vi "VI Tree.vi"   [LabVIEW 2017, in "Agilent E4980.lvlib"]
doc: "This is the instrument driver for the Agilent E4980. The VI Tree displays all the user-callable VIs of the instrument driver in an organized table."
uses:
  Agilent E4980.lvlib
  Action-Status/Clear Comparator Bin (Limit).vi
  Utility/Configure System (Display).vi
  Data/Low Level/Read Functional Data (AC Monitor).vi
panel:
  # "(c) 2007-2015 National Instruments.  ALL RIGHTS RESERVED."
  # "SEE DIAGRAM\nFOR VI TREE."
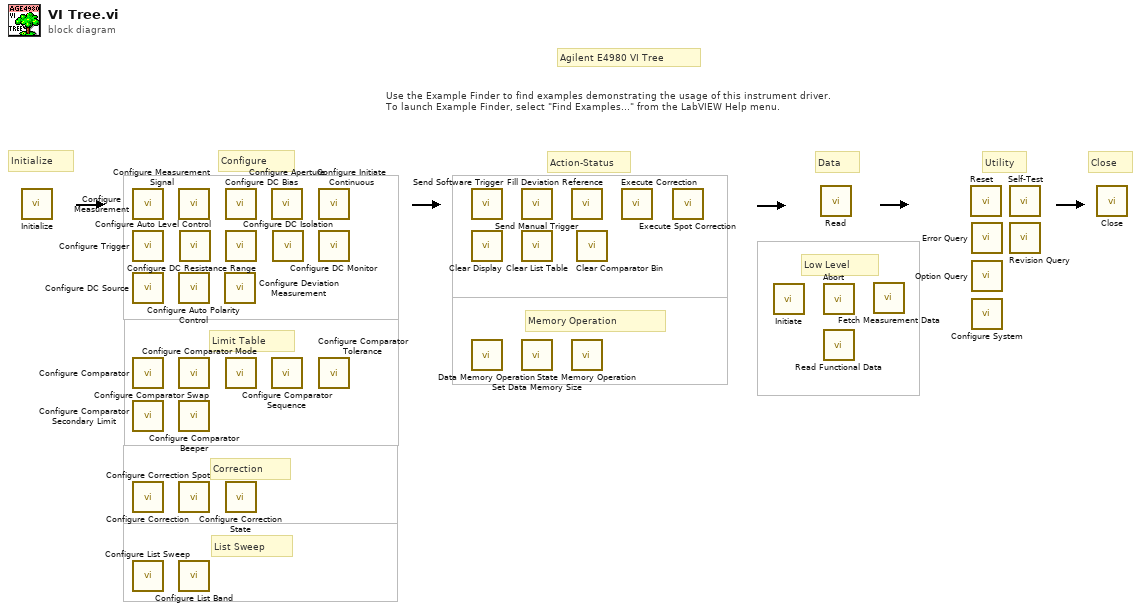
[diagram p0: block diagram]
diagram:
  # "Data"
  # "Low Level"
  # "Memory Operation"
  # "List Sweep"
  # "Correction"
  # "Limit Table"
  # "Close"
  # "Utility"
  # "Action-Status"
  # "Configure"
  # "Initialize"
  # "Agilent E4980 VI Tree"
  # "Use the Example Finder to find examples demonstrating the usage of this instrument driver.\nTo launch Example Finder, select \"Find Examples...\" from the LabVIEW Help menu."
  n1 = call "Initialize.vi"() -> ()  [unwired: 10 in, 2 out]
  n2 = call "Configure Measurement.vi"() -> ()  [unwired: 10 in, 2 out]
  n3 = call "Configure Trigger.vi"() -> ()  [unwired: 10 in, 2 out]
  n4 = call "Configure DC Source.vi"() -> ()  [unwired: 10 in, 2 out]
  n5 = call "Configure Comparator.vi"() -> ()  [unwired: 10 in, 2 out]
  n6 = call "Configure Comparator Secondary Limit.vi"() -> ()  [unwired: 10 in, 2 out]
  n7 = call "Configure Correction.vi"() -> ()  [unwired: 10 in, 2 out]
  n8 = call "Configure List Sweep.vi"() -> ()  [unwired: 10 in, 2 out]
  n9 = call "Configure Measurement Signal.vi"() -> ()  [unwired: 10 in, 2 out]
  n10 = call "Configure Auto Polarity Control.vi"() -> ()  [unwired: 10 in, 2 out]
  n11 = call "Configure Comparator Swap.vi"() -> ()  [unwired: 10 in, 2 out]
  n12 = call "Configure Comparator Beeper.vi"() -> ()  [unwired: 10 in, 2 out]
  n13 = call "Configure Correction Spot.vi"() -> ()  [unwired: 10 in, 2 out]
  n14 = call "Configure List Band.vi"() -> ()  [unwired: 10 in, 2 out]
  n15 = call "Configure Auto Level Control.vi"() -> ()  [unwired: 10 in, 2 out]
  n16 = call "Configure Deviation Measurement.vi"() -> ()  [unwired: 10 in, 2 out]
  n17 = call "Configure DC Bias.vi"() -> ()  [unwired: 10 in, 2 out]
  n18 = call "Configure DC Resistance Range.vi"() -> ()  [unwired: 10 in, 2 out]
  n19 = call "Configure Comparator Mode.vi"() -> ()  [unwired: 10 in, 2 out]
  n20 = call "Configure Correction State.vi"() -> ()  [unwired: 10 in, 2 out]
  n21 = call "Configure Aperture.vi"() -> ()  [unwired: 10 in, 2 out]
  n22 = call "Configure Comparator Sequence.vi"() -> ()  [unwired: 10 in, 2 out]
  n23 = call "Configure DC Isolation.vi"() -> ()  [unwired: 10 in, 2 out]
  n24 = call "Configure Initiate Continuous.vi"() -> ()  [unwired: 10 in, 2 out]
  n25 = call "Configure DC Monitor.vi"() -> ()  [unwired: 10 in, 2 out]
  n26 = call "Configure Comparator Tolerance.vi"() -> ()  [unwired: 10 in, 2 out]
  n27 = call "Send Software Trigger.vi"() -> ()  [unwired: 10 in, 2 out]
  n28 = call "Clear Display.vi"() -> ()  [unwired: 10 in, 2 out]
  n29 = call "Data Memory Operation.vi"() -> ()  [unwired: 10 in, 2 out]
  n30 = call "Send Manual Trigger.vi"() -> ()  [unwired: 10 in, 2 out]
  n31 = call "Clear List Table.vi"() -> ()  [unwired: 10 in, 2 out]
  n32 = call "Set Data Memory Size.vi"() -> ()  [unwired: 10 in, 2 out]
  n33 = call "Fill Deviation Reference.vi"() -> ()  [unwired: 10 in, 2 out]
  n34 = call "State Memory Operation.vi"() -> ()  [unwired: 10 in, 2 out]
  n35 = call-poly "Clear Comparator Bin.vi"() -> ()  [unwired: 10 in, 2 out]
  n36 = call "Execute Correction.vi"() -> ()  [unwired: 10 in, 2 out]
  n37 = call "Execute Spot Correction.vi"() -> ()  [unwired: 10 in, 2 out]
  n38 = call "Initiate.vi"() -> ()  [unwired: 10 in, 2 out]
  n39 = call "Read.vi"() -> ()  [unwired: 8 in, 4 out]
  n40 = call "Abort.vi"() -> ()  [unwired: 10 in, 2 out]
  n41 = call-poly "Read Functional Data.vi"() -> ()  [unwired: 8 in, 4 out]
  n42 = call "Fetch Measurement Data.vi"() -> ()  [unwired: 7 in, 5 out]
  n43 = call "Reset.vi"() -> ()  [unwired: 10 in, 2 out]
  n44 = call "Error Query.vi"() -> ()  [unwired: 8 in, 4 out]
  n45 = call "Option Query.vi"() -> ()  [unwired: 9 in, 3 out]
  n46 = call-poly "Configure System.vi"() -> ()  [unwired: 10 in, 2 out]
  n47 = call "Self-Test.vi"() -> ()  [unwired: 8 in, 4 out]
  n48 = call "Revision Query.vi"() -> ()  [unwired: 8 in, 4 out]
  n49 = call "Close.vi"() -> ()  [unwired: 11 in, 1 out]
